vi "PH_Class.ProcCases.vi"(0 "i ref in":refnum<vi>, 1 "selector":string, 2 "Data":T1, 3 "call cluster":T2={"Object"="", "Selector"="", "CallType"=enum."synchronous", "Async Object"="", "Async Selector"="", "Data Descriptor"="", "Data"=[], "Error #"=0, "Expire"=0}, 5 "error in (no error)":errorcluster) -> (14 "i ref out":refnum<vi>, 17 "answer cluster":T2={"Object"="", "Selector"="", "CallType"=enum."synchronous", "Async Object"="", "Async Selector"="", "Data Descriptor"="", "Data"=[], "Error #"=0, "Expire"=0}, 19 "error out":errorcluster)   [LabVIEW 2014, in "PH_Class.lvlib"]
doc: "This method is called by a process from within the default case in the event loop. The methods of a class that are linked to events will be called from THIS method. Add your code here."
uses:
  CS_Core/CSSystem/CoreDefs/CoreDefs.call_type.ctl
  CS_Core/BaseProcess/BaseProcess.descriptor string definition.ctl
  CS_Core/CSSystem/CoreDefs/CoreDefs.rawDataType.ctl
  CS_Core/CSSystem/CoreLib/CoreLib.string 2 byte array.vi
  CS_Core/CSSystem/CoreLib/CoreLib.byte array 2 short.vi
  PH_Class.lvlib
  CS_Core/BaseProcess/BaseProcess.lvlib
  CS_Core/CSSystem/CoreLib/CoreLib.lvlib
  CS_Core/CSObj/CSObj.lvlib
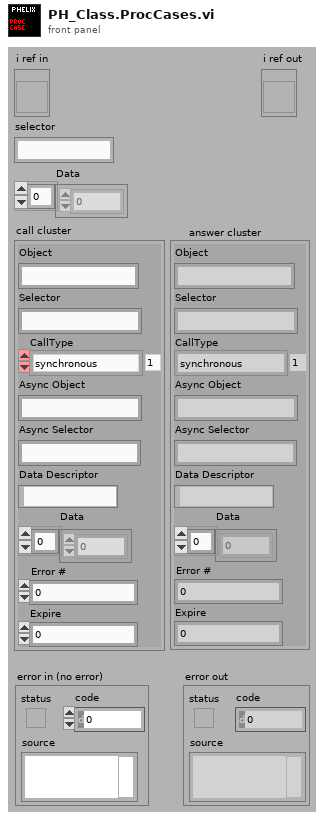
[diagram p1: front panel]
types:
  T1 = typedef "CoreDefs.rawDataType.ctl" = i8[]
  T2 = typedef "CoreDefs.call_type.ctl" = cluster{"Object":string, "Selector":string, "CallType":enum16{"simple", "synchronous", "asynchronous"}, "Async Object":string, "Async Selector":string, "Data Descriptor":T3, "Data":T1, "Error #":i32, "Expire":u32}
  T3 = typedef "BaseProcess.lvlib/BaseProcess.descriptor string definition.ctl" = string
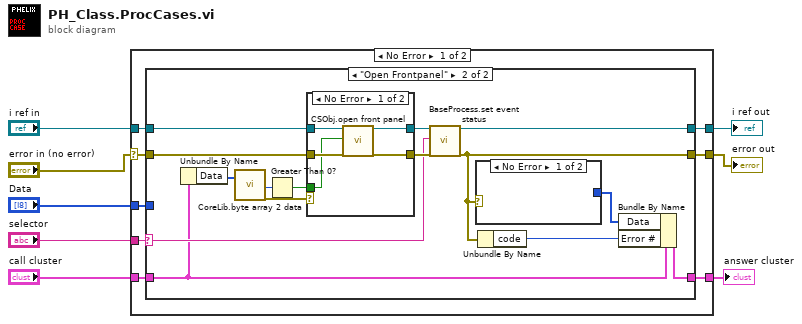
[diagram p0: block diagram]
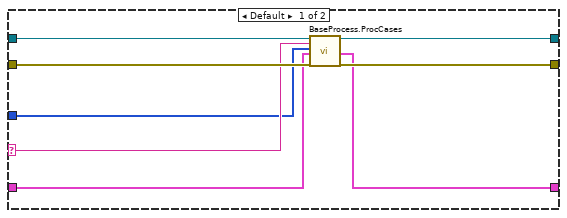
[diagram p2: hidden frame]
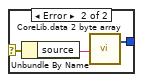
[diagram p3: hidden frame]
diagram:
  n1 = case shown="No Error" "error in (no error)" {
    selector: "error in (no error)" -> [w9 w51]
    tunnel: "selector" -> [w16 _]
    tunnel: [w15 w50] -> w7
    tunnel: "call cluster" -> [w14 w50]
    tunnel: "i ref in" -> [w13 w52]
    tunnel: [w12 w52] -> w4
    tunnel: [w11 w51] -> w3
    tunnel: "Data" -> [w10 _]
    frame No Error {
      n2 = case shown="\"Open Frontpanel\"" w16 {
        selector: w16 -> [w19 w30]
        tunnel: w10 -> [w17 _]
        tunnel: w13 -> [w18 w38]
        tunnel: [w24 w33] -> w12
        tunnel: w14 -> [w20 w27]
        tunnel: [w21 w31] -> w15
        tunnel: w9 -> [w23 w39]
        tunnel: [w22 w32] -> w11
        frame Default {
          n3 = call "BaseProcess.ProcCases.vi"("i ref in"=w18, "selector"=w19, "Data"=w17, "call cluster"=w20, "error in (no error)"=w23) -> ("i ref out"=w24:refnum<vi>, "answer cluster"=w21:T2, "error out"=w22:errorcluster)  [unwired: 12 in]
        }
        frame "Open Frontpanel" {
          n4 = Unbundle By Name(w27) -> ("Data"=w28:T1)
          n5 = call-poly "CoreLib.byte array 2 data.vi"("byteArray"=w28) -> ("i16"=w29:i16, "error out"=w26:errorcluster)  [unwired: 16 in, 1 out]
          n6 = Greater Than 0?(x=w29) -> (x > 0?=w25:bool)
          n7 = case shown="No Error" w26 {
            tunnel: [w46 w49] -> w35
            tunnel: [w44 w48] -> w34
            tunnel: w38 -> [w47 w49]
            tunnel: w39 -> [w45 w48]
            tunnel: w25 -> [w43 _]
            frame No Error {
              n8 = call "CSObj.open front panel.vi"("i ref in"=w47, "frontPanelOpen"=w43, "error in (no error)"=w45) -> ("i ref out"=w46:refnum<vi>, "error out"=w44:errorcluster)  [unwired: 15 in]
            }
            frame Error {
            }
          }
          n9 = call "BaseProcess.set event status.vi"("i ref in"=w35, "EventStatus"=w30, "error in (no error)"=w34) -> ("i ref out"=w33:refnum<vi>, "error out"=w32:errorcluster)  [unwired: 14 in, 1 out]
          n10 = case shown="No Error" w32 {
            selector: w32 -> [_ w42]
            tunnel: [_ w40] -> w36
            frame No Error {
            }
            frame Error {
              n11 = Unbundle By Name(w42) -> ("source"=w41:string)
              n12 = call-poly "CoreLib.data 2 byte array.vi"("string"=w41) -> ("byteArray out"=w40:T1)  [unwired: 18 in]
            }
          }
          n13 = Unbundle By Name(w32) -> ("code"=w37:i32)
          n14 = Bundle By Name(cluster=w27, "Data"=w36, "Error #"=w37) -> (w31:T2)
        }
      }
    }
    frame Error {
    }
  }
  "answer cluster" <- w7
  "i ref out" <- w4
  "error out" <- w3
